vi "Test-Trigger.vi"() -> ()   [LabVIEW 2020]
uses:
  g_industrial_cam/Camera/Camera.lvclass
  g_industrial_cam/Camera/Set Value (String).vi
  g_industrial_cam/Camera/Get Value (Boolean).vi
panel:
  out "ID":string
  in  "stop":bool
  out "Trigger Source Read Loop":i32
  out "Trigger Source Value":bool
  out "Current Trigger Source":string
  out "error out":errorcluster
  out "Trigger Sources":string[](array[string])
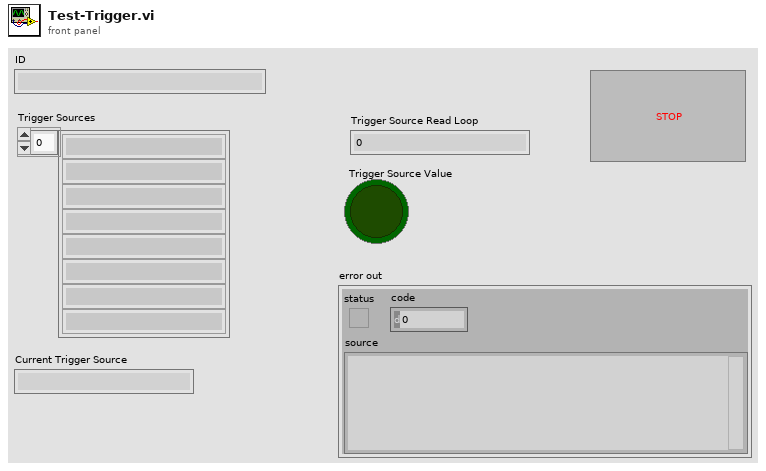
[diagram p1: front panel]
types:
  T1 = typedef "Device Enumeration.ctl" = cluster{"ID":string, "Protocol":string, "Vendor":string, "Model":string, "Serial":string, "Address":string}
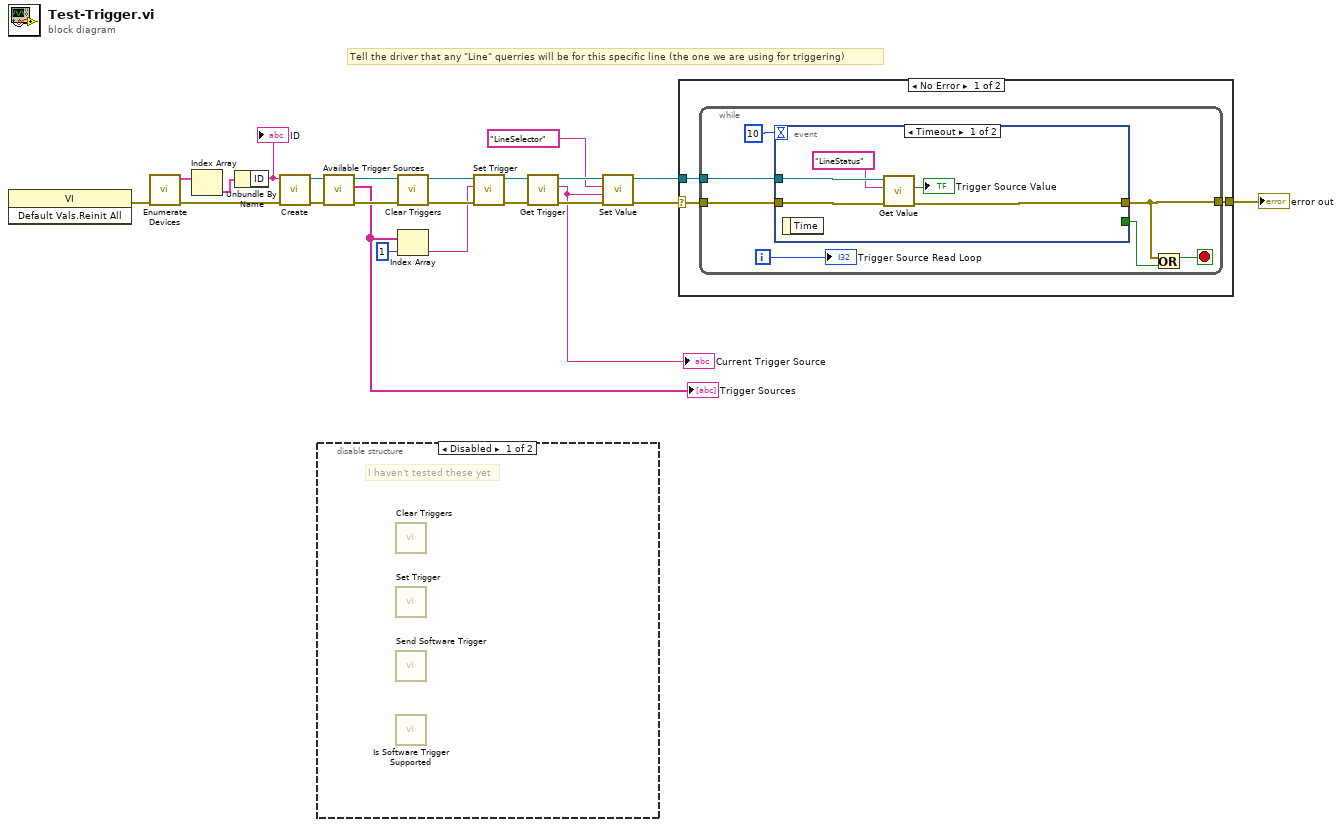
[diagram p0: block diagram]
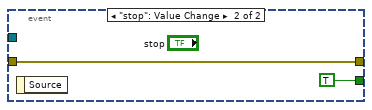
[diagram p3: hidden frame]
diagram:
  # "Tell the driver that any \"Line\" querries will be for this specific line (the one we are using for triggering)"
  n1 = invoke class="VI" method="Default Vals.Reinit All"() -> (error out=w12:errorcluster)  [unwired: 3 in, 2 out]
  n2 = call "Enumerate Devices.vi"("error in (no error)"=w12) -> ("error out"=w22:errorcluster, "Devices"=w23:T1[])  [unwired: 9 in]
  n3 = Index Array(array=w23) -> (element=w21:T1)  [unwired: 1 in]
  n4 = Unbundle By Name(w21) -> ("ID"=w20:string)
  "ID" <- w20
  n5 = call "Create.vi"("error in (no error)"=w22, "Identifier (ID, IP etc)"=w20) -> ("error out"=w5:errorcluster, "Camera"=w6:refnum<class "Camera.lvclass">)  [unwired: 8 in]
  n6 = disable-structure shown="Disabled" {
    frame Disabled {
      # "I haven't tested these yet"
      n7 = call "Clear Triggers.vi"() -> ()  [unwired: 10 in, 2 out]
      n8 = call "Set Trigger.vi"() -> ()  [unwired: 10 in, 2 out]
      n9 = call "Send Software Trigger.vi"() -> ()  [unwired: 10 in, 2 out]
      n10 = call "Is Software Trigger Supported.vi"() -> ()  [unwired: 9 in, 3 out]
    }
    frame Enabled {
    }
  }
  n11 = call "Available Trigger Sources.vi"("error in (no error)"=w5, "Camera in"=w6) -> ("error out"=w4:errorcluster, "Available Trigger Sources"=w2:string[], "Camera"=w3:refnum<class "Camera.lvclass">)  [unwired: 7 in]
  "Trigger Sources" <- w2
  n12 = call "Clear Triggers.vi"("error in (no error)"=w4, "Camera in"=w3) -> ("error out"=w9:errorcluster, "Camera"=w8:refnum<class "Camera.lvclass">)  [unwired: 8 in]
  n13 = Index Array(array=w2, index=1) -> (element=w7:string)
  n14 = call "Set Trigger.vi"("error in (no error)"=w9, "Source"=w7, "Camera in"=w8) -> ("error out"=w11:errorcluster, "Camera"=w10:refnum<class "Camera.lvclass">)  [unwired: 7 in]
  n15 = call "Get Trigger.vi"("error in (no error)"=w11, "Camera in"=w10) -> ("error out"=w19:errorcluster, "Trigger Source"=w13:string, "Camera"=w16:refnum<class "Camera.lvclass">)  [unwired: 7 in]
  "Current Trigger Source" <- w13
  n16 = call-poly "Set Value.vi"("error in (no error)"=w19, "Value"=w13, "Name"="LineSelector", "Camera in"=w16) -> ("error out"=w17:errorcluster, "Camera"=w15:refnum<class "Camera.lvclass">)  [unwired: 6 in]
  n17 = case shown="No Error" w17 {
    selector: w17 -> [w25 w41]
    tunnel: w15 -> [w26 _]
    tunnel: [w24 w41] -> w18
    frame No Error {
      n18 = while {
        tunnel: w26 -> [w33]
        tunnel: w25 -> [w31]
        tunnel: [w30] -> w24
        i -> [w29]
        stop <- w28 stop-if-true
        n19 = event shown="[0] Timeout" {
          selector: _ -> [_ _]
          dyn-events: _ -> [_ _]
          timeout: 10 -> [_ _]
          tunnel: w33 -> [w38 _]
          tunnel: [w37 w40] -> w30
          tunnel: w31 -> [w36 w40]
          tunnel: [_ TRUE] -> w27
          event Timeout {
            n20 = event-data() -> ()  [unwired: 1 in, 1 out]
            n21 = call-poly "Get Value.vi"("error in (no error)"=w36, "Name"="LineStatus", "Camera in"=w38) -> ("error out"=w37:errorcluster, "Value"=→"Trigger Source Value":bool)  [unwired: 6 in, 1 out]
          }
          event "stop": Value Change {
            n22 = event-data() -> ()  [unwired: 1 in, 1 out]
          }
        }
        n23 = Or(x=w30, y=w27) -> (x .or. y?=w28:bool)
        "Trigger Source Read Loop" <- w29
      }
    }
    frame Error {
    }
  }
  "error out" <- w18
